vi "RSZVB Correction Manager.vi"(7 "Load Parameter (\"\")":string, 8 "error in (no error)":errorcluster {"code" format="%.0x"}, 9 "File Name (\"D:\\\\user\\\\data\")":string="D:\\user\\data" caption="File Name (\"D:\\user\\data\")", 10 "Operation To Be Performed (Load)":i32(ring) items=["Load", "Store"], 11 "VISA session":refnum<visa-resource-name>) -> (0 "error out":errorcluster {"code" format="%.0x"}, 3 "dup VISA session":refnum<visa-resource-name>)   [LabVIEW 2011]
doc: "This VI provides operations which allows to loads trace data from a specified power meter correction file or trace file and assigns it to a trace with a specified name. Traces are created using the CALCulate<Ch>:PARameter:SDEFine... command. Or saves the current power loss list to a specified power meter correction list file.\n\nRemote-control command(s):\nMMEMory:STORe:CORRection:TCOefficient '<file name>'\nMMEMory:LOAD:CORRection:TCOefficient '<file name>'[,'<parameter\nname/trace name>']"
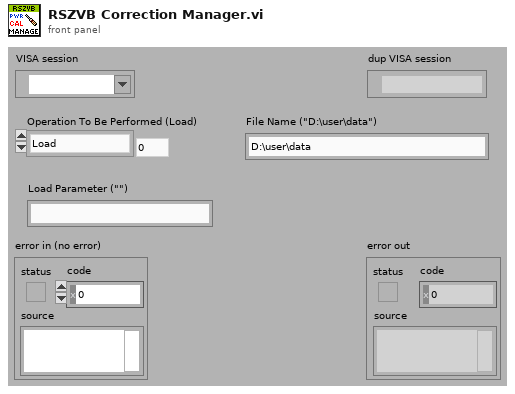
[diagram p1: front panel]
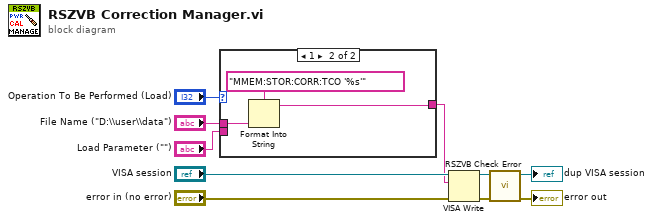
[diagram p0: block diagram]
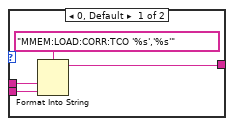
[diagram p2: hidden frame]
diagram:
  n1 = case shown="1" "Operation To Be Performed (Load)" {
    tunnel: "File Name (\"D:\\\\user\\\\data\")" -> [w13 w16]
    tunnel: "Load Parameter (\"\")" -> [w12 _]
    tunnel: [w11 w15] -> w1
    frame 0, Default {
      n2 = Format Into String(format string="MMEM:LOAD:CORR:TCO '%s','%s'", w13, w12) -> (resulting string=w11:string)  [unwired: 2 in, 1 out]
    }
    frame 1 {
      n3 = Format Into String(format string="MMEM:STOR:CORR:TCO '%s'", w16) -> (resulting string=w15:string)  [unwired: 2 in, 1 out]
    }
  }
  n4 = VISA Write(VISA resource name="VISA session", write buffer=w1, error in (no error)="error in (no error)") -> (VISA resource name out=w6:refnum<visa-resource-name>, error out=w7:errorcluster)  [unwired: 1 out]
  n5 = call "RSZVB Check Error.vi"("error in (no error)"=w7, "VISA session"=w6) -> ("error out"=→"error out":errorcluster, "dup VISA session"=→"dup VISA session":refnum<visa-resource-name>)  [unwired: 8 in]
